vi "Deploy and wait.vi"(8 "error in (no error)":errorcluster, 10 "UUT Path":path, 11 "WorkspaceManager in":T1) -> (0 "error out":errorcluster, 2 "UUT Path dup":path, 3 "WorkspaceManager out":T1)   [LabVIEW 2020]
uses:
  <vilib>/NI VeriStand/Execution/Workspace/WorkspaceAPI.ctl
  NationalInstruments.VeriStand.ClientAPI
  <vilib>/nisyscfg/Close (System).vi
  <vilib>/NI VeriStand/Execution/Workspace/NI_VS Workspace ExecutionAPI.lvlib
  <vilib>/nisyscfg/nisyscfg.lvlib
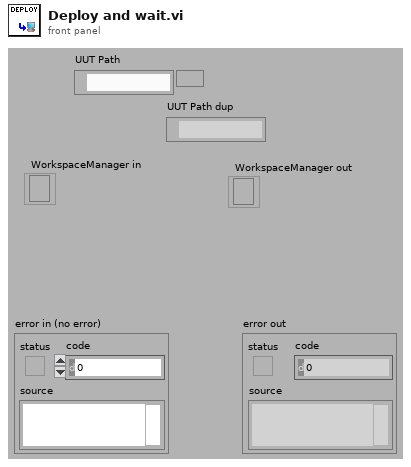
[diagram p1: front panel]
types:
  T1 = typedef "NI_VS Workspace ExecutionAPI.lvlib/WorkspaceAPI.ctl" = refnum<k24>
  T2 = typedef "NI_VS Workspace ExecutionAPI.lvlib/SystemState.ctl" = u8
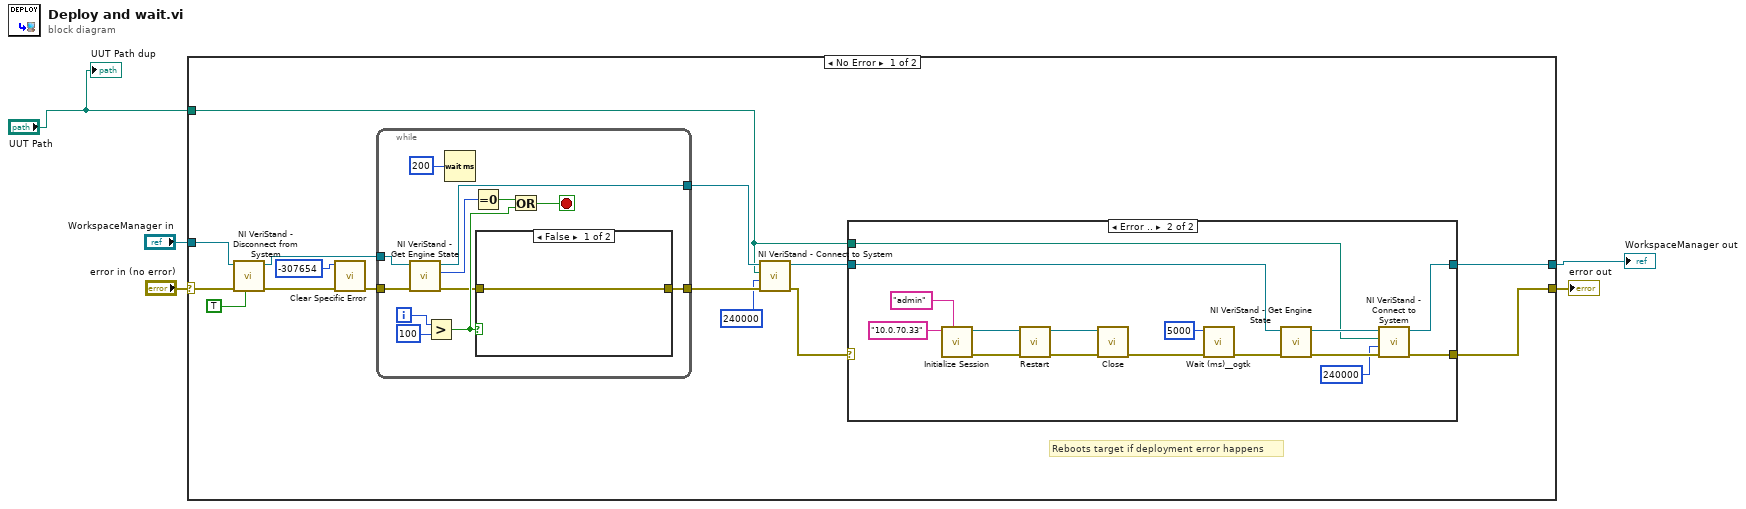
[diagram p0: block diagram]
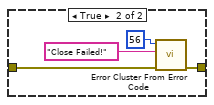
[diagram p3: hidden frame]
diagram:
  n1 = case shown="No Error" "error in (no error)" {
    selector: "error in (no error)" -> [w18 w57]
    tunnel: [w10 w57] -> w5
    tunnel: [w7 w56] -> w4
    tunnel: "WorkspaceManager in" -> [w17 w56]
    tunnel: "UUT Path" -> [w6 _]
    frame No Error {
      # "Reboots target if deployment error happens"
      n2 = call <vilib>:"NI VeriStand - Disconnect from System.vi"("Undeploy System Definition (F)"=TRUE, "error in (no error)"=w18, "WorkspaceManager in"=w17) -> ("error out"=w14:errorcluster, "WorkspaceManager out"=w16:T1)  [unwired: 7 in]
      n3 = call "Clear Specific Error.vi"("error in (no error)"=w14, "code"=-307654) -> ("error out"=w13:errorcluster)  [unwired: 8 in, 1 out]
      n4 = while {
        tunnel: w13 -> [w50]
        tunnel: w16 -> [w49]
        tunnel: [w39] -> w19
        tunnel: [w48] -> w20
        i -> [w45]
        stop <- w42 stop-if-true
        n5 = call <vilib>:"NI VeriStand - Get Engine State.vi"("error in (no error)"=w50, "WorkspaceManager in"=w49) -> ("error out"=w40:errorcluster, "System State"=w46:T2, "WorkspaceManager  out"=w48:T1)  [unwired: 4 in, 3 out]
        n6 = Greater?(x=w45, y=100) -> (0:w41:bool)
        n7 = Wait (ms)(milliseconds to wait=u32 200) -> ()  [unwired: 1 out]
        n8 = Equal To 0?(x=w46) -> (x = 0?=w43:bool)
        n9 = case shown="False" w41 {
          tunnel: [w51 w54] -> w39
          tunnel: w40 -> [w51 w55]
          frame False {
          }
          frame True {
            n10 = call <vilib>:"Error Cluster From Error Code.vi"("error in (no error)"=w55, "error message (\"\")"="Close Failed!" ("error message (\"\")"), "error code (0)"=56) -> ("error out"=w54:errorcluster)  [unwired: 6 in]
          }
        }
        n11 = Or(x=w43, y=w41) -> (x .or. y?=w42:bool)
      }
      n12 = call <vilib>:"NI VeriStand - Connect to System.vi"("error in (no error)"=w19, "Timeout (60000 ms)"=u32 240000, "System Definition File (.nivssdf)"=w6, "WorkspaceManager in"=w20) -> ("error out"=w9:errorcluster, "WorkspaceManager out"=w8:T1)  [unwired: 6 in]
      n13 = case shown="Error .." w9 {
        selector: w9 -> [w21 _]
        tunnel: [w21 w26] -> w10
        tunnel: w8 -> [w22 w31]
        tunnel: [w22 w25] -> w7
        tunnel: w6 -> [_ w28]
        frame No Error {
        }
        frame Error {
          n14 = call <vilib>:"Initialize Session.vi"("User Name"="admin", "Target (localhost)"="10.0.70.33") -> ("error out"=w36:errorcluster, "Session out"=w35:refnum<k21>)  [unwired: 8 in]
          n15 = call <vilib>:"Restart.vi"("error in (no error)"=w36, "Session in"=w35) -> ("error out"=w34:errorcluster, "Session out"=w33:refnum<k21>)  [unwired: 7 in, 1 out]
          n16 = call-poly <vilib>:"Close.vi"("error in (no error)"=w34, "Session in"=w33) -> ("error out"=w32:errorcluster)  [unwired: 9 in]
          n17 = call <userlib>:"Wait (ms)__ogtk.vi"("error in (no error)"=w32, "milliseconds to wait"=u32 5000) -> ("error out"=w24:errorcluster)  [unwired: 8 in, 1 out]
          n18 = call <vilib>:"NI VeriStand - Get Engine State.vi"("error in (no error)"=w24, "WorkspaceManager in"=w31) -> ("error out"=w30:errorcluster, "WorkspaceManager  out"=w29:T1)  [unwired: 4 in, 4 out]
          n19 = call <vilib>:"NI VeriStand - Connect to System.vi"("error in (no error)"=w30, "Timeout (60000 ms)"=u32 240000, "System Definition File (.nivssdf)"=w28, "WorkspaceManager in"=w29) -> ("error out"=w26:errorcluster, "WorkspaceManager out"=w25:T1)  [unwired: 6 in]
        }
      }
    }
    frame Error {
    }
  }
  "error out" <- w5
  "WorkspaceManager out" <- w4
  "UUT Path dup" <- "UUT Path"
